vi "ListDevices.vi"(8 "error in (no error)":errorcluster) -> (0 "error out":errorcluster, 1 "Serial Numbers":string[](array[string]), 2 "Product Names":string[](array[string]), 3 "Vendors":string[](array[string]))   [LabVIEW 2016, in "Instrument.lvclass"]
uses:
  levylab_inst/lvsrc/SMOs/Instrument/Instrument.lvclass
  <vilib>/nisyscfg/Close (System).vi
  <vilib>/nisyscfg/nisyscfg.lvlib
  <resource>/objmgr/nicriosae.rc
panel:
  out "Simulated?":string[](array[string])
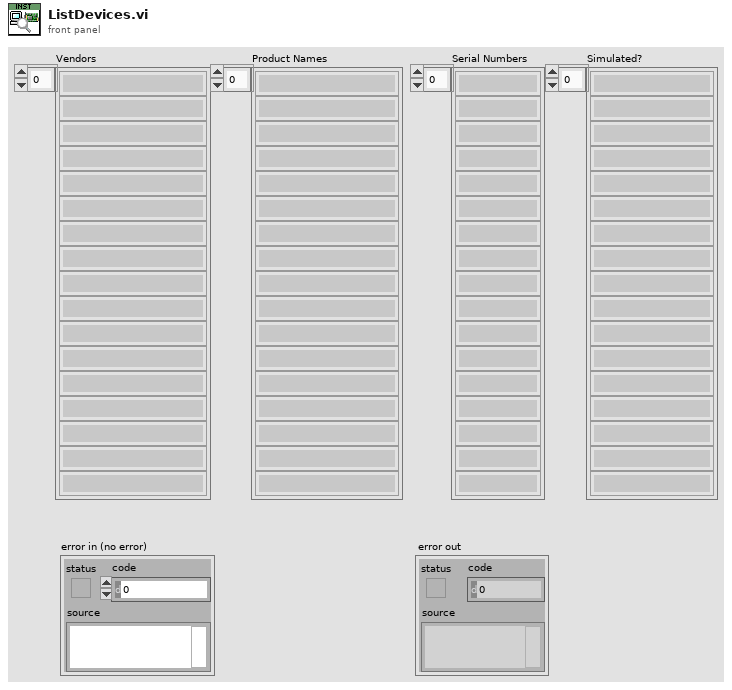
[diagram p1: front panel]
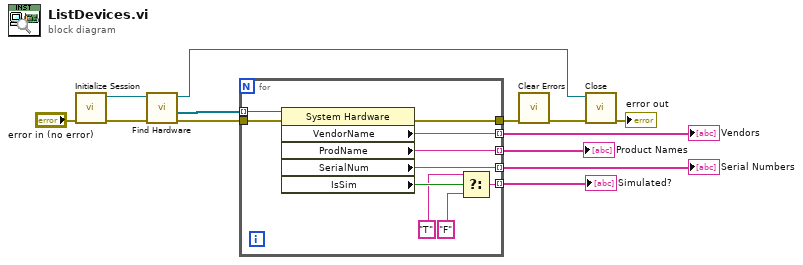
[diagram p0: block diagram]
diagram:
  n1 = call <vilib>:"Initialize Session.vi"("error in (no error)"="error in (no error)") -> ("error out"=w12:errorcluster, "Session out"=w13:refnum<k21>)  [unwired: 9 in]
  n2 = call <vilib>:"Find Hardware.vi"("error in (no error)"=w12, "Session in"=w13) -> ("error out"=w5:errorcluster, "Resources out"=w11:refnum<k20>[], "Session out"=w3:refnum<k21>)  [unwired: 6 in, 1 out]
  n3 = for {
    tunnel: w11 -> [w23] mode=indexing
    tunnel: [w22] -> w6
    tunnel: [w21] -> w10 mode=indexing
    tunnel: [w20] -> w9 mode=indexing
    tunnel: [w19] -> w8 mode=indexing
    tunnel: [w15] -> w7 mode=indexing
    tunnel: w5 -> [w14]
    n4 = property class="System Hardware"(reference=w23, error in=w14) -> (error out=w22:errorcluster, "VendorName"=w21:string, "ProdName"=w20:string, "SerialNum"=w19:string, "IsSim"=w18:bool)  [unwired: 1 out]
    n5 = Select(t="T" ("Devices & Chassis:Serial Number"), s=w18, f="F" ("Devices & Chassis:Serial Number")) -> (s? t:f=w15:string)
  }
  "Vendors" <- w10
  "Product Names" <- w9
  "Serial Numbers" <- w8
  "Simulated?" <- w7
  n6 = call <vilib>:"Clear Errors.vi"("error in (no error)"=w6) -> ("error out"=w4:errorcluster)  [unwired: 5 in, 1 out]
  n7 = call-poly <vilib>:"Close.vi"("error in (no error)"=w4, "Session in"=w3) -> ("error out"=→"error out":errorcluster)  [unwired: 9 in]
